vi "Test Weekdays.vi"(8 "error in":errorcluster) -> (0 "error out":errorcluster)   [LabVIEW 2013]
uses:
  source/formatter.iso8601/DateTime.ISO8601.lvclass
  source/formatter.iso8601/ISO8601 Date Formats.ctl
  source/formatter.iso8601/DateTime.ISO8601.lvclass/DateTime.ISO8601.ctl
  source/formatter.iso8601/Timestamp to ISO8601 Day.vi
  source/isLeapYear (timestamp).vi
  source/formatter.iso8601/Timestamp to ISO8601 Year.vi
  source/isLeapYear (integer).vi
  <vilib>/addons/_JKI Toolkits/Caraya/classes/Assert/Assert Equal Value_Variant.vi
  <vilib>/addons/_JKI Toolkits/Caraya/classes/Assert/Assert True.vi
  <vilib>/addons/_JKI Toolkits/Caraya/classes/Test/Test.lvclass
  <vilib>/addons/_JKI Toolkits/Caraya/classes/Assert/Assert.lvclass
  source/formatter/DateTimeFormatter.lvclass
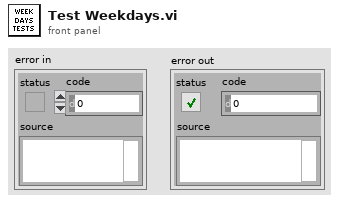
[diagram p1: front panel]
types:
  T1 = typedef "ISO8601 Date Formats.ctl" = enum16{"UTC Date-Time", "ISO Time", "Date", "Calendar Month", "Week", "Week-Day", "Month-Day", "Ordinal Date"}
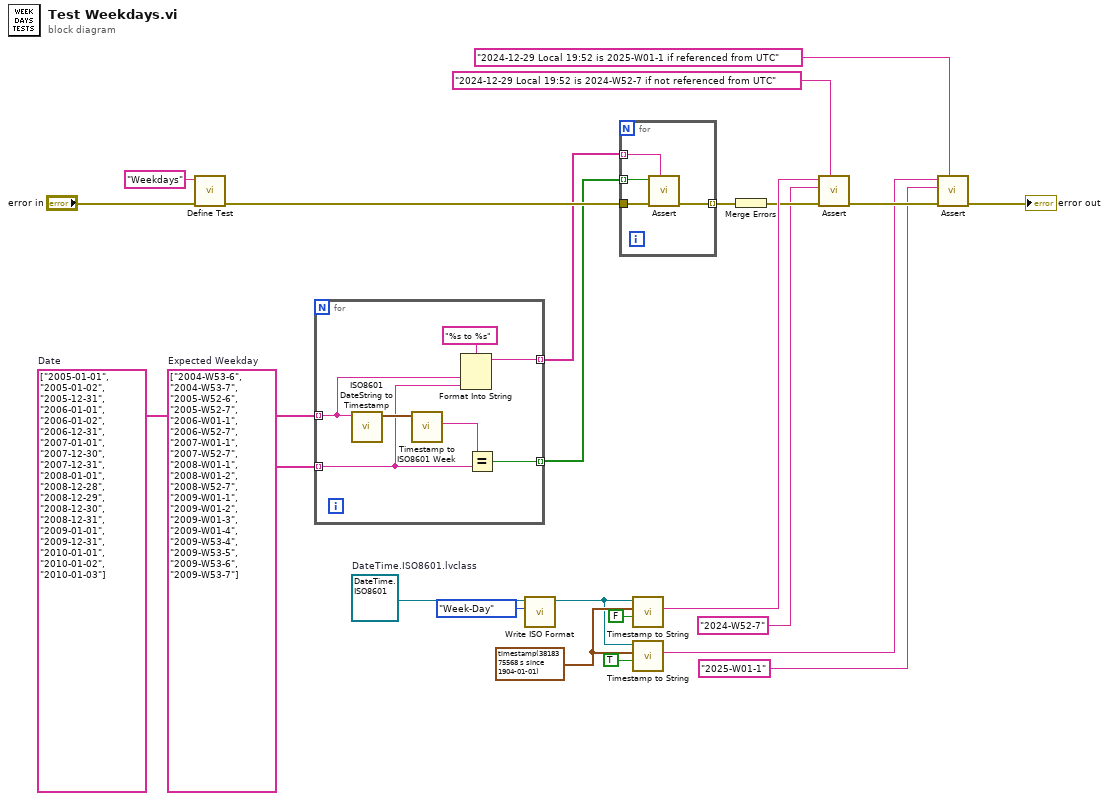
[diagram p0: block diagram]
diagram:
  w11 = timestamp(3818375568.3080063 s since 1904-01-01) ("current time")
  w14 = refnum<class "DateTime.ISO8601.lvclass"> refnum  # DateTime.ISO8601.lvclass
  w20 = string[] ["2005-01-01", "2005-01-02", "2005-12-31", "2006-01-01", "2006-01-02", "2006-12-31", "2007-01-01", "2007-12-30", "2007-12-31", "2008-01-01", "2008-12-28", "2008-12-29", "2008-12-30", "2008-12-31", "2009-01-01", "2009-12-31", "2010-01-01", "2010-01-02", "2010-01-03"]  # Date
  w21 = string[] ["2004-W53-6", "2004-W53-7", "2005-W52-6", "2005-W52-7", "2006-W01-1", "2006-W52-7", "2007-W01-1", "2007-W52-7", "2008-W01-1", "2008-W01-2", "2008-W52-7", "2009-W01-1", "2009-W01-2", "2009-W01-3", "2009-W01-4", "2009-W53-4", "2009-W53-5", "2009-W53-6", "2009-W53-7"]  # Expected Weekday
  n1 = call <vilib>:"Define Test.vi"("error in (no error)"="error in", "Label (VI Title)"="Weekdays") -> ("error out"=w19:errorcluster)  [unwired: 8 in, 1 out]
  n2 = for {
    tunnel: w21 -> [w28] mode=indexing
    tunnel: w20 -> [w26] mode=indexing
    tunnel: [w25] -> w17 mode=indexing
    tunnel: [w24] -> w16 mode=indexing
    n3 = call "ISO8601 DateString to Timestamp.vi"("ISO8601 Date String"=w26) -> ("Timestamp"=w29:timestamp)  [unwired: 8 in, 2 out]
    n4 = call "Timestamp to ISO8601 Week.vi"("Timestamp (now)"=w29) -> ("ISO8601 Weekday"=w30:string)  [unwired: 8 in, 2 out]
    n5 = Format Into String(format string="%s to %s" ("Label (VI Title)"), w26, w28) -> (resulting string=w25:string)  [unwired: 2 in, 1 out]
    n6 = Equal?(x=w30, y=w28) -> (x = y?=w24:bool)
  }
  n7 = call "Write ISO Format.vi"("ISO Format"=ISO8601_Date_Formats."Week-Day", "DateTime.ISO8601 in"=w14) -> ("DateTime.ISO8601 out"=w10:refnum<class "DateTime.ISO8601.lvclass">)  [unwired: 9 in]
  n8 = for {
    tunnel: w19 -> [w34]
    tunnel: [w33] -> w18 mode=indexing
    tunnel: w17 -> [w32] mode=indexing
    tunnel: w16 -> [w31] mode=indexing
    n9 = call-poly <vilib>:"Assert.vi"("Label"=w32, "error in (no error)"=w34, "True?"=w31) -> ("error out"=w33:errorcluster)  [unwired: 7 in, 1 out]
  }
  n10 = call "Timestamp to String.vi"("UTC? (F)"=FALSE, "Timestamp (now)"=w11, "DateTimeFormatter in"=w10) -> ("DateTime String"=w9:string)  [unwired: 6 in, 2 out]
  n11 = call "Timestamp to String.vi"("UTC? (F)"=TRUE, "Timestamp (now)"=w11, "DateTimeFormatter in"=w10) -> ("DateTime String"=w5:string)  [unwired: 6 in, 2 out]
  n12 = Merge Errors(w18) -> (w8:errorcluster)
  n13 = call-poly <vilib>:"Assert.vi"("Label"="2024-12-29 Local 19:52 is 2024-W52-7 if not referenced from UTC" ("x"), "error in (no error)"=w8, "Y"="2024-W52-7" ("x"), "X"=w9) -> ("error out"=w7:errorcluster)  [unwired: 6 in, 1 out]
  n14 = call-poly <vilib>:"Assert.vi"("Label"="2024-12-29 Local 19:52 is 2025-W01-1 if referenced from UTC" ("x"), "error in (no error)"=w7, "Y"="2025-W01-1" ("x"), "X"=w5) -> ("error out"=→"error out":errorcluster)  [unwired: 6 in, 1 out]
